vi "TestCounter.Reset.vi"(8 "error in":errorcluster) -> (0 "error out":errorcluster, 2 "TestCount":u64, 5 "TestCount path":path)   [LabVIEW 2019, in "Tools.lvlib"]
uses:
  Tools.lvlib
  ProjectPaths.ctl
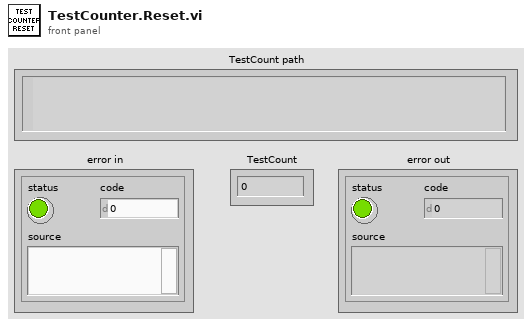
[diagram p1: front panel]
types:
  T1 = typedef "Tools.lvlib/ProjectPaths.ctl" = enum16{"Settings dir", "Logs dir", "Resources dir", "Verification file", "Users file", "Root dir"}
  T2 = enum16{"open", "replace", "create", "open or create", "replace or create", "replace or create with confirmation"}
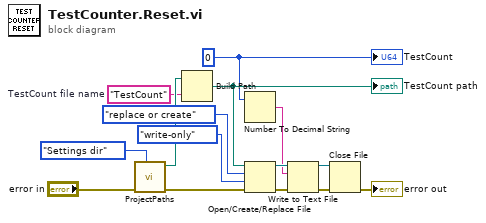
[diagram p0: block diagram]
diagram:
  w2 = u64 0 ("number")
  w12 = "TestCount"  # TestCount file name
  n1 = call "ProjectPaths.vi"("Item"=ProjectPaths."Settings dir", "Error In"="error in") -> ("Error Out"=w8:errorcluster, "Path"=w13:path)  [unwired: 8 in]
  n2 = Build Path(base path=w13, name or relative path=w12) -> (appended path=w11:path)
  "TestCount path" <- w11
  n3 = Number To Decimal String(number=w2) -> (decimal integer string=w3:string)  [unwired: 1 in]
  n4 = Open/Create/Replace File(file path (use dialog)=w11, error in=w8, operation (0:open)=T2."replace or create", access (0:read/write)=enum16{"read/write", "read-only", "write-only"}."write-only") -> (refnum out=w15:refnum<file>, error out=w14:errorcluster)  [unwired: 2 in, 1 out]
  n5 = Write to Text File(file (use dialog)=w15, text=w3, error in=w14) -> (refnum out=w5:refnum<file>, error out=w4:errorcluster)  [unwired: 1 in, 1 out]
  n6 = Close File(refnum=w5, error in=w4) -> (error out=→"error out":errorcluster)  [unwired: 1 out]
  "TestCount" <- w2
